vi "SynapseAPI-Get Known Subjects.vi"(0 "URL":string="http://localhost:24414", 11 "error in (no error)":errorcluster) -> (8 "subjects":string[](array[string]), 15 "error out":errorcluster)   [LabVIEW 2020]
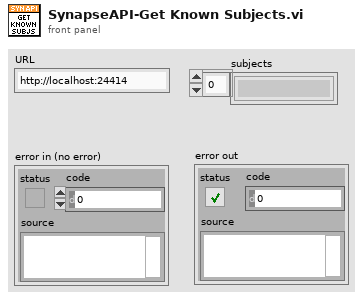
[diagram p1: front panel]
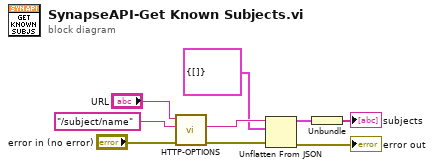
[diagram p0: block diagram]
diagram:
  n1 = call "HTTP-OPTIONS.vi"("error in (no error)"="error in (no error)", "req"="/subject/name", "URL"="URL") -> ("error out"=w6:errorcluster, "body"=w5:string)  [unwired: 6 in, 1 out]
  n2 = Unflatten From JSON(JSON string=w5, type and defaults=cluster{"subjects":string[]} {"subjects"=[]}, error in (no error)=w6) -> (value=w2:cluster{"subjects":string[]}, error out=→"error out":errorcluster)  [unwired: 4 in]
  n3 = Unbundle(w2) -> ("subjects"=→"subjects":string[])
